vi "stackVertically.vi"(4 "spacing":u16, 6 "useControlBodyOnly":bool, 7 "horizontalAlignment":T1=enum."AlignLeft", 8 "error in (no error)":errorcluster, 11 "refs":refnum<vi>[](array[refnum])) -> (0 "error out":errorcluster, 3 "refs(dup)":refnum<vi>[](array[refnum]))   [LabVIEW 2023]
doc: "Arranges the input controls vertically according to their order in the array, using the specified spacing.\nThe horizontal position is defined by the input 'horizontalAlignment'."
uses:
  Ctrls/alignment.ctl
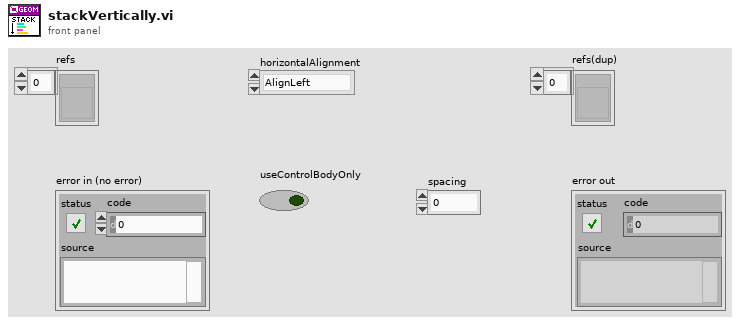
[diagram p1: front panel]
types:
  T1 = typedef "alignment.ctl" = enum16{"None", "AlignTop", "AlignBottom", "AlignHorizontalCenters", "AlignLeft", "AlignRight", "AlignVerticalCenters"}
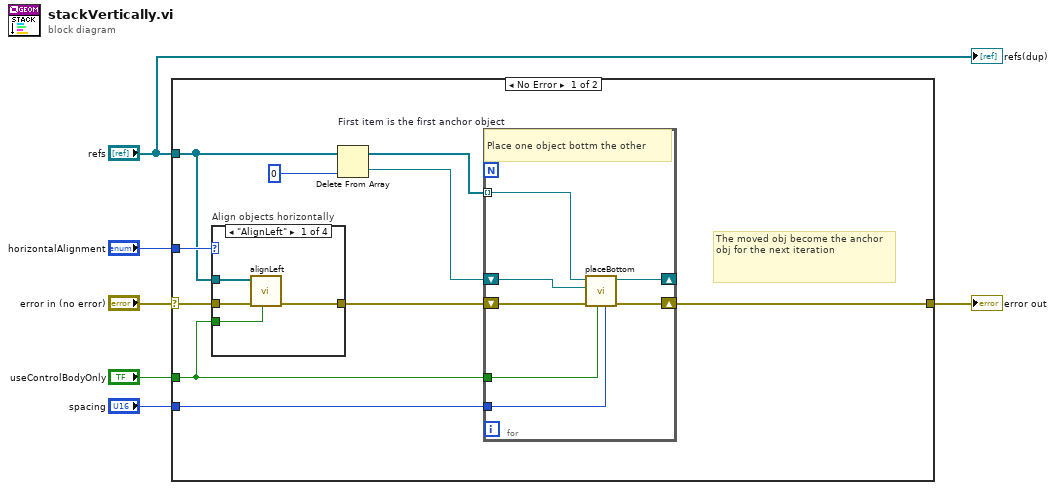
[diagram p0: block diagram]
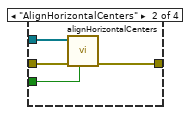
[diagram p2: hidden frame]
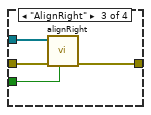
[diagram p3: hidden frame]
diagram:
  n1 = case shown="No Error" "error in (no error)" {
    selector: "error in (no error)" -> [w11 w37]
    tunnel: [w16 w37] -> w3
    tunnel: "refs" -> [w7 _]
    tunnel: "useControlBodyOnly" -> [w8 _]
    tunnel: "spacing" -> [w12 _]
    tunnel: "horizontalAlignment" -> [w9 _]
    frame No Error {
      # "The moved obj become the anchor obj for the next iteration"
      n2 = case "Align objects horizontally" shown="\"AlignLeft\"" w9 {
        tunnel: w11 -> [w20 w24 w28 w29]
        tunnel: [w19 w23 w27 w29] -> w10
        tunnel: w8 -> [w18 w22 w26 _]
        tunnel: w7 -> [w17 w21 w25 _]
        frame "AlignLeft" {
          n3 = call "alignLeft.vi"("useControlBodyOnly"=w18, "error in (no error)"=w20, "refs"=w17) -> ("error out"=w19:errorcluster)  [unwired: 7 in, 1 out]
        }
        frame "AlignHorizontalCenters" {
          n4 = call "alignHorizontalCenters.vi"("useControlBodyOnly"=w22, "error in (no error)"=w24, "refs"=w21) -> ("error out"=w23:errorcluster)  [unwired: 7 in, 1 out]
        }
        frame "AlignRight" {
          n5 = call "alignRight.vi"("useControlBodyOnly"=w26, "error in (no error)"=w28, "refs"=w25) -> ("error out"=w27:errorcluster)  [unwired: 7 in, 1 out]
        }
        frame "None", Default {
        }
      }
      n6 = Delete From Array "First item is the first anchor object"(array=w7, index=0) -> (deleted portion=w14:refnum<vi>, array with subset deleted=w13:refnum<vi>[])  [unwired: 1 in]
      n7 = for {
        shift-right: [w35] -> w16
        shift-left: w10 -> [w36]
        tunnel: w13 -> [w31] mode=indexing
        tunnel: w8 -> [w34]
        tunnel: w12 -> [w33]
        shift-right: [w30] -> _
        shift-left: w14 -> [w32]
        # "Place one object bottm the other"
        n8 = call "placeBottom.vi"("spacing"=w33, "useControlBodyOnly"=w34, "error in (no error)"=w36, "anchorObject"=w32, "movingObject"=w31) -> ("error out"=w35:errorcluster, "movingObject(dup)"=w30:refnum<vi>)  [unwired: 4 in, 1 out]
      }
    }
    frame Error {
    }
  }
  "error out" <- w3
  "refs(dup)" <- "refs"
